vi "DSF.Engine.Transfer.Create.vi"(4 "size":u64, 5 "id":i32, 6 "group offset":u64, 7 "channel blocks":T1[](array[typedef]) {"buffer offset" format="%d bytes"}, 8 "error in (no error)":errorcluster, 9 "String Buffer":refnum<class "DSF.Engine.Memory.Buffer.lvclass">, 10 "Intermediate Buffer":refnum<class "DSF.Engine.Pointer.DBL.lvclass">, 11 "Inline Buffer":refnum<class "DSF.Engine.Pointer.DBL.lvclass">) -> (0 "error out":errorcluster, 3 "Transfer out":refnum<class "DSF.Engine.Transfer.lvclass">)   [LabVIEW 2017, in "Data Sharing Framework Engine.lvlib" / "DSF.Engine.Transfer.lvclass"]
uses:
  DSF.Engine.Transfer.lvclass
  Buffer/DSF.Engine.Memory.Buffer.lvclass
  Pointer/DSF.Engine.Pointer.DBL.lvclass
  Shared/Typedefs/DSF Runtime Channel Block.ctl
  DSF Configuration API/1.0.0/Public/Controls/DSF Data Type.ctl
  DSF.Engine.Transfer.lvclass/DSF.Engine.Transfer.ctl
  Source/Data Sharing Framework Core/Engine/Data Sharing Framework Engine.lvlib
  DSF Configuration API/1.0.0/DSF Configuration API.lvlib
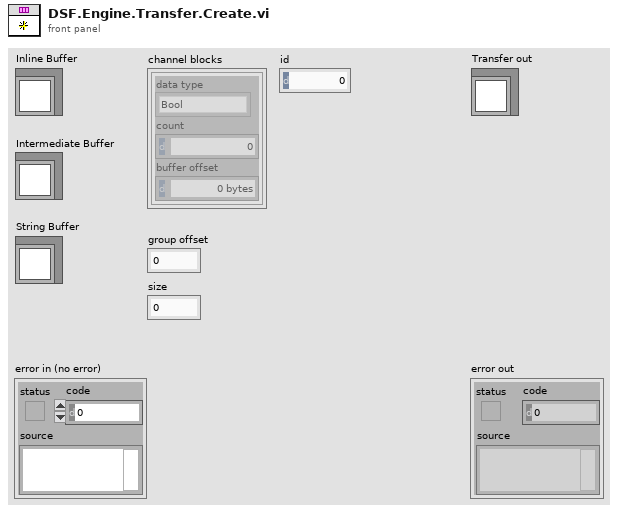
[diagram p1: front panel]
types:
  T1 = typedef "Data Sharing Framework Engine.lvlib/DSF Runtime Channel Block.ctl" = cluster{"data type":T2, "count":u64, "buffer offset":u64}
  T2 = typedef "DSF Configuration API.lvlib/DSF Data Type.ctl" = enum8{"Bool", "SGL", "DBL", "I8", "I16", "I32", "I64", "U8", "U16", "U32", "U64"}
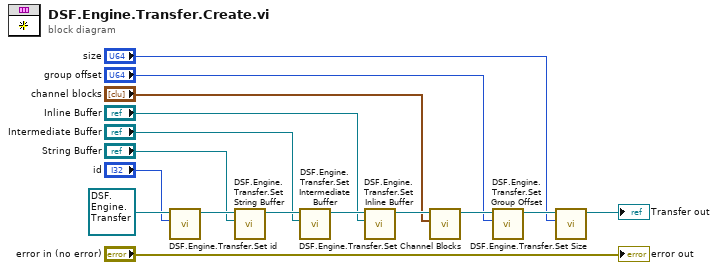
[diagram p0: block diagram]
diagram:
  n1 = call "DSF.Engine.Transfer.Set id.vi"("id"="id", "Transfer in"=refnum<class "DSF.Engine.Transfer.lvclass"> refnum) -> ("Transfer out"=w16:refnum<class "DSF.Engine.Transfer.lvclass">)  [unwired: 9 in]
  n2 = call "DSF.Engine.Transfer.Set String Buffer.vi"("Buffer"="String Buffer", "Transfer in"=w16) -> ("Transfer out"=w15:refnum<class "DSF.Engine.Transfer.lvclass">)  [unwired: 9 in]
  n3 = call "DSF.Engine.Transfer.Set Intermediate Buffer.vi"("DBL Buffer"="Intermediate Buffer", "Transfer in"=w15) -> ("Transfer out"=w14:refnum<class "DSF.Engine.Transfer.lvclass">)  [unwired: 9 in]
  n4 = call "DSF.Engine.Transfer.Set Inline Buffer.vi"("Inline Buffer"="Inline Buffer", "Transfer in"=w14) -> ("Transfer out"=w7:refnum<class "DSF.Engine.Transfer.lvclass">)  [unwired: 9 in]
  n5 = call "DSF.Engine.Transfer.Set Channel Blocks.vi"("channel blocks"="channel blocks", "Transfer in"=w7) -> ("Transfer out"=w5:refnum<class "DSF.Engine.Transfer.lvclass">)  [unwired: 9 in]
  n6 = call "DSF.Engine.Transfer.Set Group Offset.vi"("group offset"="group offset", "Transfer in"=w5) -> ("Transfer out"=w4:refnum<class "DSF.Engine.Transfer.lvclass">)  [unwired: 9 in]
  n7 = call "DSF.Engine.Transfer.Set Size.vi"("engine size"="size", "Transfer in"=w4) -> ("Transfer out"=→"Transfer out":refnum<class "DSF.Engine.Transfer.lvclass">)  [unwired: 9 in]
  "error out" <- "error in (no error)"
